vi "HTTP PUT.vi"(8 "error in (no error)":errorcluster caption="에러 입력(에러 없음)", 10 "url":string, 11 "참조 번호 입력":T1 caption="클라이언트 핸들") -> (0 "에러 출력":errorcluster, 3 "참조 번호 출력":T1 caption="클라이언트 핸들 출력")   [LabVIEW 2022 SP3]
uses:
  <vilib>/httpClient/ClientHandle.ctl
  <vilib>/httpClient/PUTBuffer.vi
  <vilib>/httpClient/LabVIEWHTTPClient.lvlib
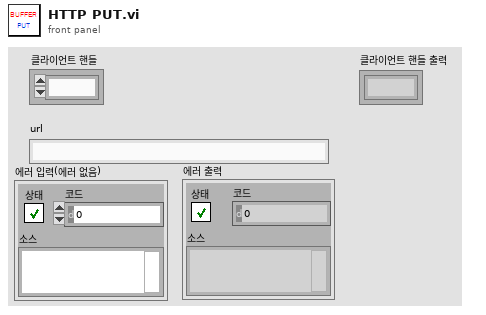
[diagram p1: front panel]
types:
  T1 = typedef "LabVIEWHTTPClient.lvlib/ClientHandle.ctl" = refnum<k1>
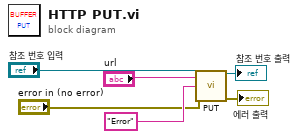
[diagram p0: block diagram]
diagram:
  n1 = call-poly <vilib>:"PUT.vi"("client handle"="참조 번호 입력", "url"="url", "buffer"="Error", "error in (no error)"="error in (no error)") -> ("client handle out"=→"참조 번호 출력":T1, "error out"=→"에러 출력":errorcluster)  [unwired: 8 in, 2 out]
